vi "JSON to Variant.vi"(8 "error in (no error)":errorcluster, 10 "Variant (Data Type)":variant, 11 "JSON Value":refnum<class "JSON Value.lvclass">) -> (0 "error out":errorcluster, 2 "Variant out":variant)   [LabVIEW 2020, in "Library Commun.lvlib" / "Variant JSON.lvlib"]
doc: "Converts a JSON value object into a LabVIEW datatype.\n\nElements in the <b>Variant (Data Type)</b> are used to retrieve information from <b>JSON Value</b>.\n\nCopyright 2012 James David Powell, Shaun Rumbell and Ton Plomp\nMore information on http://lavag.org/topic/16217-cr-json-labview"
uses:
  Variant JSON.lvlib
  JSON Value/JSON Value.lvclass
  JSON Object/JSON Object.lvclass
  JSON Value/Get as JSON string.vi
  JSON Scalar/Get as I32.vi
  JSON Scalar/Get as I64.vi
  JSON Scalar/Get as U32.vi
  JSON Scalar/Get as U64.vi
  JSON Scalar/Get as SGL.vi
  JSON Scalar/Get as DBL.vi
  JSON Scalar/Get as EXT.vi
  JSON Scalar/Get as Boolean.vi
  JSON Value/Get Item by name array.vi
  JSON Scalar/Get as Path.vi
  JSON Scalar/Get as Timestamp.vi
  <userlib>/_OpenG.lib/lvdata/lvdata.llb/openg_variant.lvlib
  JSON Scalar/JSON Scalar.lvclass
  Get Polymorphic/JSON GetSet.lvlib
  <vilib>/Utility/VariantDataType/VariantType.lvlib
  support/JSON support.lvlib
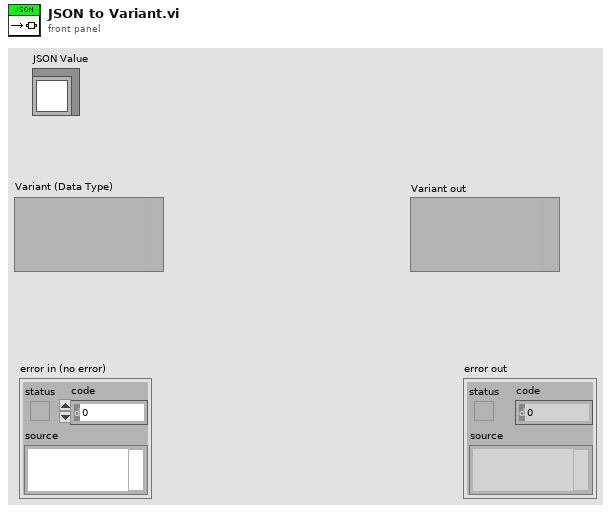
[diagram p1: front panel]
types:
  T1 = typedef "VariantType.lvlib/Type.ctl" = enum8{"Invalid Type", "Void", "I8", "I16", "I32", "I64", "U8", "U16", "U32", "U64", "Single Float", "Double Float", "Extended Float", "Single Complex", "Double Complex", "Extended Complex", "Enum U8", "Enum U16", "Enum U32", "Enum U64", "Single Float With Unit", "Double Float With Unit", "Extended Float With Unit", "Single Complex with Unit", "Double Complex with Unit", "Extended Complex with Unit", "Boolean", "String", "Path", "Picture", "Tag", "Array", "Cluster", "Variant", "LV Variant", "Waveform", "Timestamp", "Digital Waveform", "Digital Data", "ExpressData", "Refnum", "External Data", "VI", "Poly VI", "LabVIEW Class Instance", "Fixed Point"}
  T2 = cluster{"[0]":variant, "[1]":variant, "[2]":variant}
  T3 = cluster{"[0]":variant, "[1]":variant, "[2]":variant, "[3]":variant}
  T4 = cluster{"[0]":variant, "[1]":variant, "[2]":variant, "[3]":variant, "[4]":variant}
  T5 = cluster{"[0]":variant, "[1]":variant, "[2]":variant, "[3]":variant, "[4]":variant, "[5]":variant}
  T6 = cluster{"[0]":variant, "[1]":variant, "[2]":variant, "[3]":variant, "[4]":variant, "[5]":variant, "[6]":variant}
  T7 = cluster{"[0]":variant, "[1]":variant, "[2]":variant, "[3]":variant, "[4]":variant, "[5]":variant, "[6]":variant, "[7]":variant}
  T8 = cluster{"[0]":variant, "[1]":variant, "[2]":variant, "[3]":variant, "[4]":variant, "[5]":variant, "[6]":variant, "[7]":variant, "[8]":variant}
  T9 = cluster{"[0]":variant, "[1]":variant, "[2]":variant, "[3]":variant, "[4]":variant, "[5]":variant, "[6]":variant, "[7]":variant, "[8]":variant, "[9]":variant}
  T10 = typedef "VariantType.lvlib/RefnumType.ctl" = enum16{"NotARefnum", "UnknownRefnum", "Generic", "Datalog", "ByteStream", "Device", "Occurence", "TCPNetConnection", "Auto", "Menu", "Imaq", "Hardware", "DataSocket", "Visa", "IVI", "UDPNetConnection", "Notifier", "Queue", "Irda", "EventReg", "DotNet", "UserEvent", "Callback", "UNUSED_EMPTY_POSITION", "BlueToothNetConnection", "LVObjApp", "LVObjVI", "LVObjUnknown", "GenericClass", "UserDefinedRefnumTag", "DataValue", "RT FIFO", "TDMS File"}
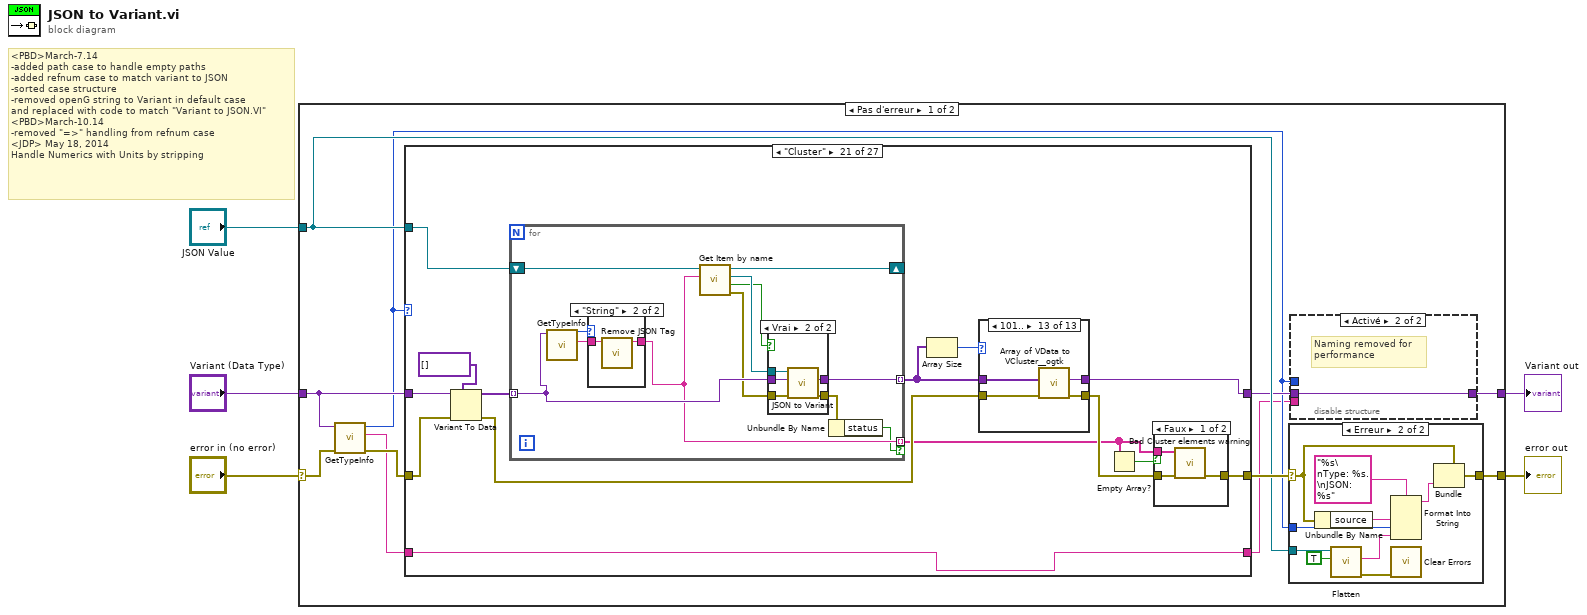
[diagram p0: block diagram]
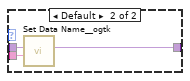
[diagram p3: hidden frame]
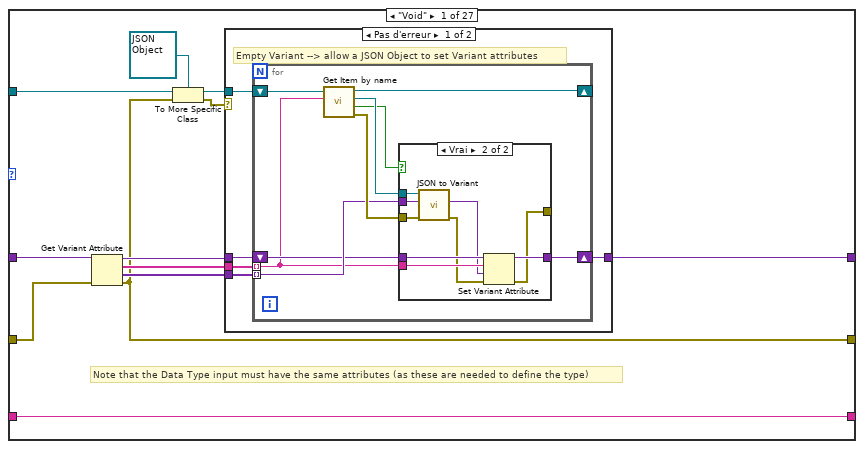
[diagram p5: hidden frame]
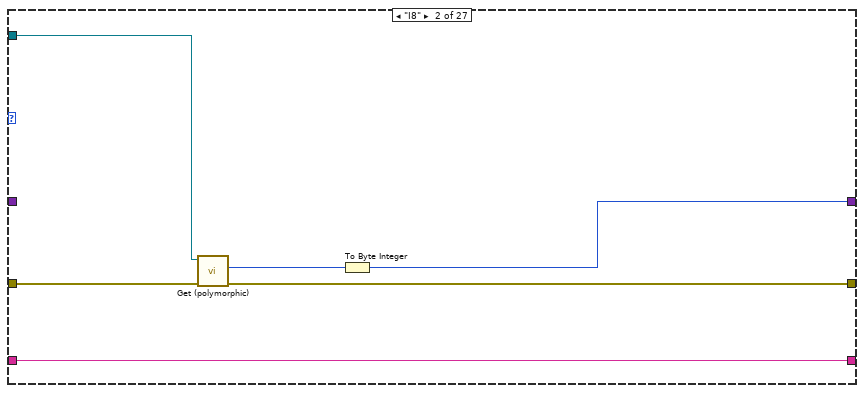
[diagram p8: hidden frame]
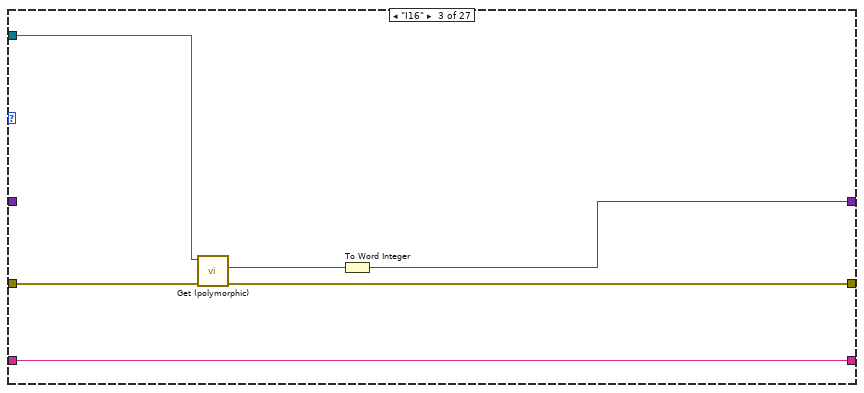
[diagram p9: hidden frame]
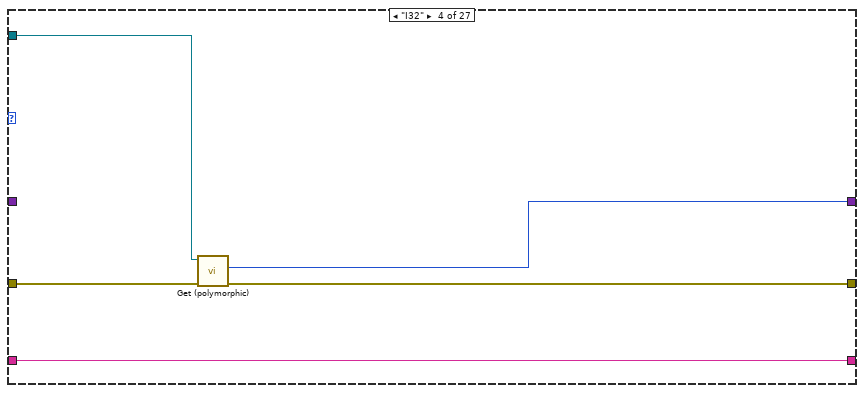
[diagram p10: hidden frame]
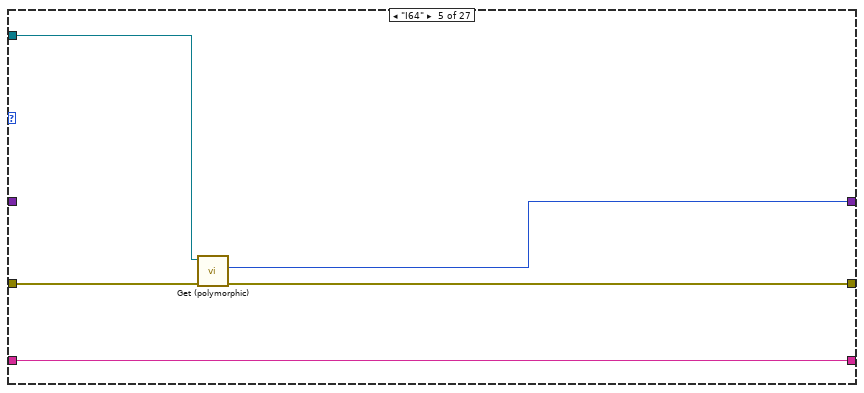
[diagram p11: hidden frame]
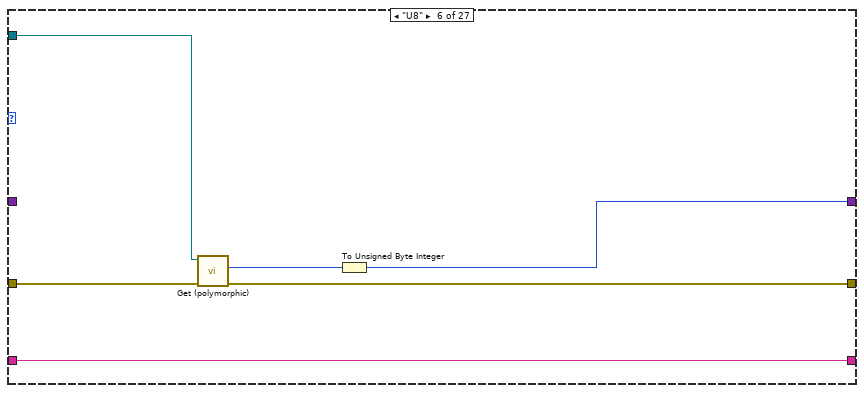
[diagram p12: hidden frame]
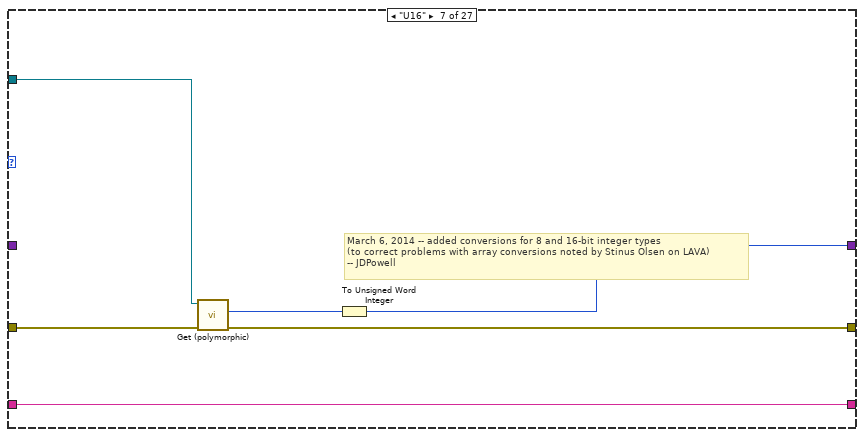
[diagram p13: hidden frame]
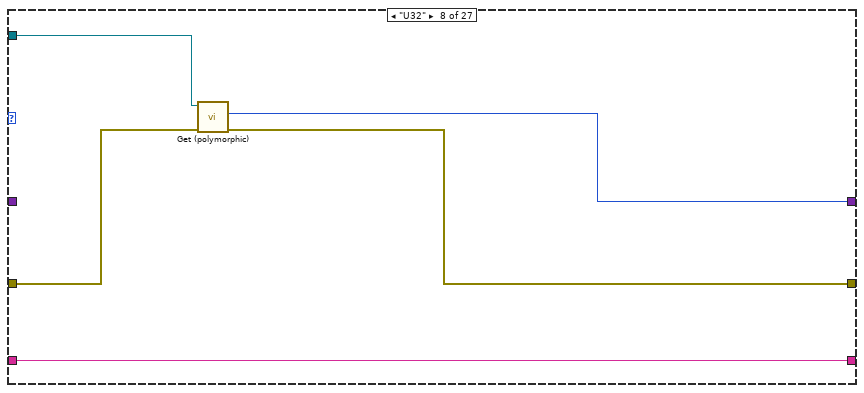
[diagram p14: hidden frame]
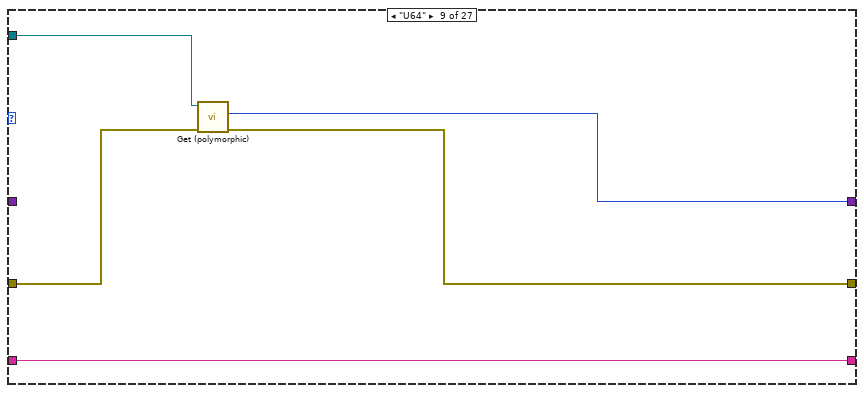
[diagram p15: hidden frame]
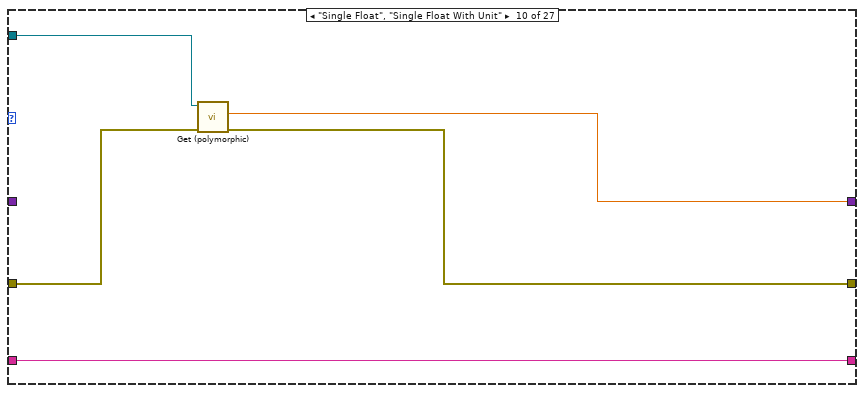
[diagram p16: hidden frame]
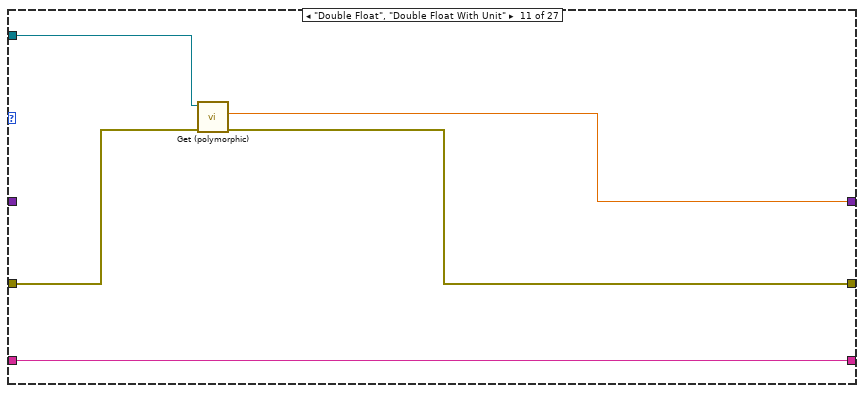
[diagram p17: hidden frame]
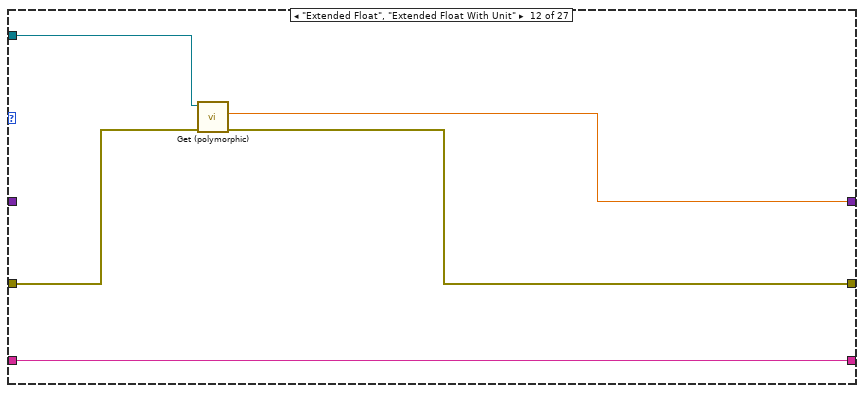
[diagram p18: hidden frame]
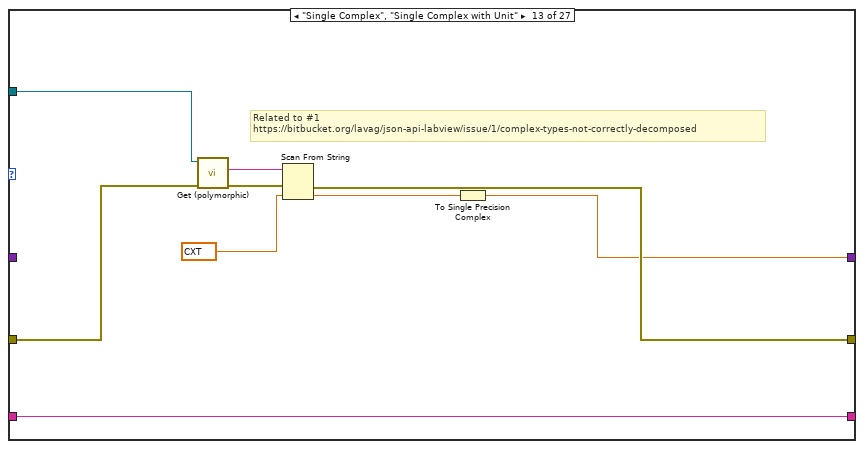
[diagram p19: hidden frame]
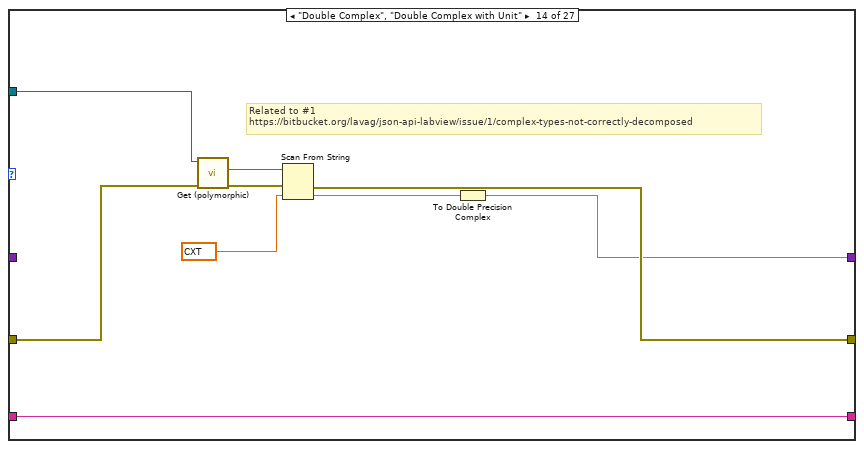
[diagram p20: hidden frame]
diagram:
  # "<PBD>March-7.14\n-added path case to handle empty paths\n-added refnum case to match variant to JSON\n-sorted case structure\n-removed openG string to Variant in default case \nand replaced with code to match \"Variant to JSON.VI\"\n<PBD>March-10.14\n-removed \"=>\" handling from refnum case\n<JDP> May 18, 2014\nHandle Numerics with Units by stripping"
  n1 = case shown="Pas d'erreur" "error in (no error)" {
    selector: "error in (no error)" -> [w10 w368]
    tunnel: [w15 w368] -> w4
    tunnel: "Variant (Data Type)" -> [w11 w367]
    tunnel: "JSON Value" -> [w14 _]
    tunnel: [w12 w367] -> w1
    frame No Error {
      n2 = call <vilib>:"GetTypeInfo.vi"("error in (no error)"=w10, "Variant"=w11) -> ("error out"=w9:errorcluster, "Name"=w7:string, "Type Enum"=w8:T1)  [unwired: 5 in, 2 out]
      n3 = case shown="\"Cluster\"" w8 {
        tunnel: w11 -> [w44 _ _ _ _ _ _ _ _ _ _ _ _ _ _ w167 _ _ _ w196 w209 w286 _ _ w304 w334 w363]
        tunnel: w9 -> [w39 w78 w84 w89 w94 w100 w106 w111 w116 w121 w126 w131 w141 w150 w158 w162 w170 w178 w192 w198 w208 w285 w291 w295 w303 _ w366]
        tunnel: [w38 w77 w83 w88 w93 w99 w105 w110 w115 w120 w125 w130 w136 w145 w153 w161 w169 w177 w191 w197 w213 w288 w290 w296 w300 w335 w361] -> w16
        tunnel: w14 -> [w48 w80 w86 w91 w96 w102 w108 w113 w118 w123 w128 w133 w142 w151 w159 w165 w172 w180 w193 w199 w212 w287 w293 w298 w302 w337 w365]
        tunnel: [w40 w76 w82 w90 w95 w98 w104 w112 w117 w122 w127 w132 w135 w144 w155 w166 w171 w179 w190 w194 w211 w280 w292 w297 w301 w336 w360] -> w13
        tunnel: w7 -> [w37 w75 w81 w87 w92 w97 w103 w109 w114 w119 w124 w129 w134 w143 w152 w160 w168 w176 w189 w195 w205 w279 w289 w294 w299 w343 w358]
        tunnel: [w37 w75 w81 w87 w92 w97 w103 w109 w114 w119 w124 w129 w134 w143 w152 w160 w168 w176 w189 w195 w205 w279 w289 w294 w299 w343 w358] -> w6
        frame "Void" {
          # "Note that the Data Type input must have the same attributes (as these are needed to define the type)"
          n4 = Get Variant Attribute(Variant=w44, error in=w39) -> (duplicate Variant=w43:variant, names=w42:string[], values=w41:variant[], error out=w38:errorcluster)  [unwired: 2 in]
          n5 = To More Specific Class(target class=refnum<class "JSON Object.lvclass"> refnum ("JSON Object in"), reference=w48, error in=w38) -> (specific class reference=w46:refnum<class "JSON Object.lvclass">, error out=w45:errorcluster)
          n6 = case shown="Pas d'erreur" w45 {
            tunnel: w46 -> [w50 _]
            tunnel: w43 -> [w51 w74]
            tunnel: w42 -> [w53 _]
            tunnel: w41 -> [w52 _]
            tunnel: [w49 w74] -> w40
            frame No Error {
              # "Empty Variant --> allow a JSON Object to set Variant attributes"
              n7 = for {
                tunnel: w53 -> [w56] mode=indexing
                tunnel: w52 -> [w58] mode=indexing
                shift-right: [w55] -> w49
                shift-left: w51 -> [w57]
                shift-right: [w54] -> _
                shift-left: w50 -> [w59]
                n8 = call-dynamic "Get Item by name.vi"("name"=w56, "JSON Object in"=w59) -> ("error out"=w62:errorcluster, "found"=w60:bool, "Value"=w61:refnum<class "JSON Value.lvclass">, "JSON Object out"=w54:refnum<class "JSON Object.lvclass">)  [unwired: 6 in]
                n9 = case shown="Vrai" w60 {
                  tunnel: w62 -> [w64 w73]
                  tunnel: [w64 w65] -> _
                  tunnel: w58 -> [_ w72]
                  tunnel: w61 -> [_ w71]
                  tunnel: w57 -> [w63 w70]
                  tunnel: w56 -> [_ w69]
                  tunnel: [w63 w68] -> w55
                  frame False {
                  }
                  frame True {
                    n10 = call "JSON to Variant.vi"("error in (no error)"=w73, "Variant (Data Type)"=w72, "JSON Value"=w71) -> ("error out"=w66:errorcluster, "Variant out"=w67:variant)  [unwired: 7 in]
                    n11 = Set Variant Attribute(Variant=w70, name=w69, value=w67, error in=w66) -> (Variant out=w68:variant, error out=w65:errorcluster)  [unwired: 1 out]
                  }
                }
              }
            }
            frame Error {
            }
          }
        }
        frame "I8" {
          n12 = call-poly "Get (polymorphic).vi"("error in (no error)"=w78, "JSON Scalar in"=w80) -> ("error out"=w77:errorcluster, "Number"=w79:i32)  [unwired: 7 in, 1 out]
          n13 = To Byte Integer(number=w79) -> (8bit integer=w76:i8)
        }
        frame "I16" {
          n14 = call-poly "Get (polymorphic).vi"("error in (no error)"=w84, "JSON Scalar in"=w86) -> ("error out"=w83:errorcluster, "Number"=w85:i32)  [unwired: 7 in, 1 out]
          n15 = To Word Integer(number=w85) -> (16bit integer=w82:i16)
        }
        frame "I32" {
          n16 = call-poly "Get (polymorphic).vi"("error in (no error)"=w89, "JSON Scalar in"=w91) -> ("error out"=w88:errorcluster, "Number"=w90:i32)  [unwired: 7 in, 1 out]
        }
        frame "I64" {
          n17 = call-poly "Get (polymorphic).vi"("error in (no error)"=w94, "JSON Scalar in"=w96) -> ("error out"=w93:errorcluster, "Number"=w95:i64)  [unwired: 7 in, 1 out]
        }
        frame "U8" {
          n18 = call-poly "Get (polymorphic).vi"("error in (no error)"=w100, "JSON Scalar in"=w102) -> ("error out"=w99:errorcluster, "Number"=w101:u32)  [unwired: 7 in, 1 out]
          n19 = To Unsigned Byte Integer(number=w101) -> (unsigned 8bit integer=w98:u8)
        }
        frame "U16" {
          # "March 6, 2014 -- added conversions for 8 and 16-bit integer types\n(to correct problems with array conversions noted by Stinus Olsen on LAVA)\n-- JDPowell"
          n20 = call-poly "Get (polymorphic).vi"("error in (no error)"=w106, "JSON Scalar in"=w108) -> ("error out"=w105:errorcluster, "Number"=w107:u32)  [unwired: 7 in, 1 out]
          n21 = To Unsigned Word Integer(number=w107) -> (unsigned 16bit integer=w104:u16)
        }
        frame "U32" {
          n22 = call-poly "Get (polymorphic).vi"("error in (no error)"=w111, "JSON Scalar in"=w113) -> ("error out"=w110:errorcluster, "Number"=w112:u32)  [unwired: 7 in, 1 out]
        }
        frame "U64" {
          n23 = call-poly "Get (polymorphic).vi"("error in (no error)"=w116, "JSON Scalar in"=w118) -> ("error out"=w115:errorcluster, "Number"=w117:u64)  [unwired: 7 in, 1 out]
        }
        frame "Single Float", "Single Float With Unit" {
          n24 = call-poly "Get (polymorphic).vi"("error in (no error)"=w121, "JSON Value in"=w123) -> ("error out"=w120:errorcluster, "Number"=w122:sgl)  [unwired: 7 in, 1 out]
        }
        frame "Double Float", "Double Float With Unit" {
          n25 = call-poly "Get (polymorphic).vi"("error in (no error)"=w126, "JSON Value in"=w128) -> ("error out"=w125:errorcluster, "Number"=w127:dbl)  [unwired: 7 in, 1 out]
        }
        frame "Extended Float", "Extended Float With Unit" {
          n26 = call-poly "Get (polymorphic).vi"("error in (no error)"=w131, "JSON Value in"=w133) -> ("error out"=w130:errorcluster, "Number"=w132:ext)  [unwired: 7 in, 1 out]
        }
        frame "Single Complex", "Single Complex with Unit" {
          # "Related to #1\nhttps://bitbucket.org/lavag/json-api-labview/issue/1/complex-types-not-correctly-decomposed"
          n27 = call-poly "Get (polymorphic).vi"("error in (no error)"=w141, "JSON Scalar in"=w142) -> ("error out"=w137:errorcluster, "LabVIEW Text"=w140:string)  [unwired: 7 in, 1 out]
          n28 = Scan From String(input string=w140, error in=w137, default 1=cxt 0.0+0.0i) -> (error out=w136:errorcluster, output 1=w138:cxt)  [unwired: 2 in, 2 out]
          n29 = To Single Precision Complex(1:w138) -> (0:w135:csg)
        }
        frame "Double Complex", "Double Complex with Unit" {
          # "Related to #1\nhttps://bitbucket.org/lavag/json-api-labview/issue/1/complex-types-not-correctly-decomposed"
          n30 = call-poly "Get (polymorphic).vi"("error in (no error)"=w150, "JSON Scalar in"=w151) -> ("error out"=w146:errorcluster, "LabVIEW Text"=w149:string)  [unwired: 7 in, 1 out]
          n31 = Scan From String(input string=w149, error in=w146, default 1=cxt 0.0+0.0i) -> (error out=w145:errorcluster, output 1=w147:cxt)  [unwired: 2 in, 2 out]
          n32 = To Double Precision Complex(1:w147) -> (0:w144:cdb)
        }
        frame "Extended Complex", "Extended Complex with Unit" {
          n33 = call-poly "Get (polymorphic).vi"("error in (no error)"=w158, "JSON Scalar in"=w159) -> ("error out"=w154:errorcluster, "LabVIEW Text"=w157:string)  [unwired: 7 in, 1 out]
          n34 = Scan From String(input string=w157, error in=w154, default 1=cxt 0.0+0.0i) -> (error out=w153:errorcluster, output 1=w155:cxt)  [unwired: 2 in, 2 out]
        }
        frame "Enum U8".."Enum U64" {
          n35 = call-poly "Get (polymorphic).vi"("error in (no error)"=w162, "JSON Scalar in"=w165) -> ("error out"=w163:errorcluster, "LabVIEW Text"=w164:string)  [unwired: 7 in, 1 out]
          n36 = call <userlib>:"Set Enum String Value__ogtk.vi"("error in (no error)"=w163, "String Value"=w164, "Default Enum Value"=w167) -> ("error out"=w161:errorcluster, "Enum"=w166:variant)  [unwired: 7 in]
        }
        frame "Boolean" {
          n37 = call-poly "Get (polymorphic).vi"("error in (no error)"=w170, "JSON Value in"=w172) -> ("error out"=w169:errorcluster, "Boolean"=w171:bool)  [unwired: 7 in, 1 out]
        }
        frame "String" {
          # "Allow marking of LabVIEW strings as representing JSON, rather than JSON strings.\nThis is to allow using Variants where some ot the subelement structure is unknown/dynamic -- JDP, April 2014"
          n38 = call "Tag for JSON Text.vi"() -> ("Tag for JSON text"=w173:string)  [unwired: 11 in]
          n39 = Match Pattern(string=w176, regular expression=w173) -> (after substring=w175:string, offset past match=w174:i32)  [unwired: 1 in, 2 out]
          n40 = case shown="0.." w174 {
            tunnel: w180 -> [w184 w188]
            tunnel: [w183 w187] -> w179
            tunnel: w178 -> [w182 w186]
            tunnel: [w181 w185] -> w177
            tunnel: w175 -> [_ _]
            frame ..-1 {
              n41 = call-poly "Get (polymorphic).vi"("error in (no error)"=w182, "JSON Scalar in"=w184) -> ("error out"=w181:errorcluster, "LabVIEW Text"=w183:string)  [unwired: 7 in, 1 out]
            }
            frame 0.. {
              n42 = call-poly "Get (polymorphic).vi"("error in (no error)"=w186, "JSON Value in"=w188) -> ("error out"=w185:errorcluster, "<JSON>"=w187:string)  [unwired: 8 in]
            }
          }
        }
        frame "Path" {
          n43 = call-poly "Get (polymorphic).vi"("error in (no error)"=w192, "JSON Scalar in"=w193) -> ("error out"=w191:errorcluster, "path"=w190:path)  [unwired: 7 in, 1 out]
        }
        frame "Array" {
          # "Dec 2015, JDP rewrite for higher speed with large arrays"
          n44 = call "Get Array as Variant.vi"("error in (no error)"=w198, "Variant (Data Type)"=w196, "JSON Value in"=w199) -> ("error out"=w197:errorcluster, "Default VData"=w194:variant)  [unwired: 7 in]
        }
        frame "Cluster" {
          n45 = Variant To Data(error in=w208, type=variant[] [], Variant=w209) -> (data=w207:variant[], error out=w206:errorcluster)
          n46 = for {
            shift-right: [w267] -> _
            shift-left: w212 -> [w268]
            tunnel: [w265] -> w202 mode=indexing
            tunnel: [w263] -> w204 mode=indexing if=w259
            tunnel: w207 -> [w264] mode=indexing
            n47 = call <vilib>:"GetTypeInfo.vi"("Variant"=w264) -> ("Name"=w258:string, "Type Enum"=w257:T1)  [unwired: 6 in, 3 out]
            n48 = case shown="\"String\"" w257 {
              tunnel: w258 -> [w269 w271]
              tunnel: [w269 w270] -> w263
              frame Default {
              }
              frame "String" {
                n49 = call "Remove JSON Tag.vi"("Name"=w271) -> ("Name (tag stripped)"=w270:string)  [unwired: 9 in, 1 out]
              }
            }
            n50 = call-dynamic "Get Item by name.vi"("name"=w263, "JSON Value In"=w268) -> ("error out"=w262:errorcluster, "found"=w260:bool, "Value"=w261:refnum<class "JSON Value.lvclass">, "JSON Value Out"=w267:refnum<class "JSON Value.lvclass">)  [unwired: 6 in]
            n51 = case shown="Vrai" w260 {
              tunnel: w262 -> [w272 w278]
              tunnel: [w272 w277] -> w266
              tunnel: w264 -> [w273 w276]
              tunnel: w261 -> [_ w275]
              tunnel: [w273 w274] -> w265
              frame False {
              }
              frame True {
                n52 = call "JSON to Variant.vi"("error in (no error)"=w278, "Variant (Data Type)"=w276, "JSON Value"=w275) -> ("error out"=w277:errorcluster, "Variant out"=w274:variant)  [unwired: 7 in]
              }
            }
            n53 = Unbundle By Name(w266) -> ("status"=w259:bool)
          }
          n54 = Array Size(array=w202) -> (size(s)=w201:i32)
          n55 = case shown="101.." w201 {
            tunnel: [variant ("VCluster") w217 w220 w223 w226 w229 w232 w235 w238 w241 w244 w247 w252] -> w211
            tunnel: [w214 w216 w219 w222 w225 w228 w231 w234 w237 w240 w243 w246 w251] -> w210
            tunnel: w206 -> [w214 w216 w219 w222 w225 w228 w231 w234 w237 w240 w243 w246 w250]
            tunnel: w202 -> [_ w218 w221 w224 w227 w230 w233 w236 w239 w242 w245 w248 w249]
            frame ..0 {
            }
            frame 1 {
              n56 = Array To Cluster(array=w218) -> (cluster=w217:cluster{"[0]":variant})
            }
            frame 2 {
              n57 = Array To Cluster(array=w221) -> (cluster=w220:cluster{"[0]":variant, "[1]":variant})
            }
            frame 3 {
              n58 = Array To Cluster(array=w224) -> (cluster=w223:T2)
            }
            frame 4 {
              n59 = Array To Cluster(array=w227) -> (cluster=w226:T3)
            }
            frame 5 {
              n60 = Array To Cluster(array=w230) -> (cluster=w229:T4)
            }
            frame 6 {
              n61 = Array To Cluster(array=w233) -> (cluster=w232:T5)
            }
            frame 7 {
              n62 = Array To Cluster(array=w236) -> (cluster=w235:T6)
            }
            frame 8 {
              n63 = Array To Cluster(array=w239) -> (cluster=w238:T7)
            }
            frame 9 {
              n64 = Array To Cluster(array=w242) -> (cluster=w241:T8)
            }
            frame 10 {
              n65 = Array To Cluster(array=w245) -> (cluster=w244:T9)
            }
            frame Default {
              n66 = call "Array of Variants to Cluster.vi"("Var"=w248) -> ("Cluster of Variants"=w247:variant)  [unwired: 10 in]
            }
            frame 101.. {
              n67 = call <userlib>:"Array of VData to VCluster__ogtk.vi"("error in (no error)"=w250, "Array"=w249) -> ("error out"=w251:errorcluster, "VCluster"=w252:variant)  [unwired: 8 in]
            }
          }
          n68 = Empty Array?(array=w204) -> (empty?=w203:bool)
          n69 = case shown="Faux" w203 {
            tunnel: [w255 w256] -> w213
            tunnel: w210 -> [w254 w256]
            tunnel: w204 -> [w253 _]
            frame False {
              n70 = call "Bad Cluster elements warning.vi"("error in (no error)"=w254, "Error items"=w253) -> ("error out"=w255:errorcluster)  [unwired: 9 in]
            }
            frame True {
            }
          }
        }
        frame "Variant", "LV Variant" {
          # "Get item inside variant, convert, and then put back in a variant"
          n71 = Variant To Data(error in=w285, type=variant, Variant=w286) -> (data=w283:variant, error out=w284:errorcluster)
          n72 = call "JSON to Variant.vi"("error in (no error)"=w284, "Variant (Data Type)"=w283, "JSON Value"=w287) -> ("error out"=w288:errorcluster, "Variant out"=w281:variant)  [unwired: 7 in]
          n73 = To Variant(anything=w281) -> (Variant=w280:variant)
        }
        frame "Waveform" {
          n74 = call "Get as Waveform.vi"("error in (no error)"=w291, "JSON Value In"=w293) -> ("error out"=w290:errorcluster, "Waveform"=w292:waveform(dbl))  [unwired: 7 in, 1 out]
        }
        frame "Timestamp" {
          n75 = call-poly "Get (polymorphic).vi"("error in (no error)"=w295, "JSON Value in"=w298) -> ("error out"=w296:errorcluster, "Time Stamp"=w297:timestamp)  [unwired: 7 in, 1 out]
        }
        frame "Refnum" {
          n76 = call-poly "Get (polymorphic).vi"("error in (no error)"=w303, "JSON Scalar in"=w302) -> ("error out"=w306:errorcluster, "LabVIEW Text"=w305:string)  [unwired: 7 in, 1 out]
          n77 = call <vilib>:"GetRefnumInfo.vi"("error in (no error)"=w306, "Variant"=w304) -> ("error out"=w307:errorcluster, "ReferenceType"=w308:T10)  [unwired: 6 in, 2 out]
          n78 = case shown="\"Visa\", \"IVI\", \"UserDefinedRefnumTag\"" w308 {
            tunnel: [w309 w318 w331] -> w301
            tunnel: w307 -> [w310 w312 w329]
            tunnel: [w310 w311 w330] -> w300
            tunnel: w305 -> [_ w313 w326]
            tunnel: w304 -> [w309 w321 w333]
            frame "NotARefnum", "UnknownRefnum" {
            }
            frame "Visa", "IVI", "UserDefinedRefnumTag" {
              n79 = Variant To Data(error in=w312, type="", Variant=w321) -> (data=w319:string, error out=w311:errorcluster)
              n80 = Scan From String(input string=w313, default 1=w319) -> (error out=w317:errorcluster, output 1=w314:string)  [unwired: 3 in, 2 out]
              n81 = Select(t="", s=w317, f=w314) -> (s? t:f=w316:string)
              n82 = To Variant(anything=w316) -> (Variant=w318:variant)
            }
            frame Default {
              w325 = 0
              n83 = Scan From String(input string=w326, default 1=w325) -> (error out=w328:errorcluster, output 1=w327:i32)  [unwired: 3 in, 2 out]
              n84 = Select(t=w325, s=w328, f=w327) -> (s? t:f=w323:i32)
              n85 = Variant To Flattened String(Variant=w333) -> (1:w332:i16[])  [unwired: 1 out]
              n86 = Type Cast(type="", x=w323) -> (*(type *) &x=w324:string)
              n87 = Flattened String To Variant(4:w329, 6:w324, 7:w332) -> (0:w330:errorcluster, 3:w331:variant)
            }
          }
        }
        frame "LabVIEW Class Instance" {
          w338 = refnum<class "JSON Value.lvclass"> refnum ("JSON Value")
          n88 = Variant To Data(type=refnum<class> refnum ("LabVIEW Object"), Variant=w334) -> (data=w339:refnum<class>, error out=w341:errorcluster)  [unwired: 1 in]
          n89 = To More Specific Class(target class=w338, reference=w339, error in=w341) -> (error out=w340:errorcluster)  [unwired: 1 out]
          n90 = case shown="Pas d'erreur" w340 {
            selector: w340 -> [w351 _]
            tunnel: w339 -> [w350 _]
            tunnel: w338 -> [w349 _]
            tunnel: w337 -> [w345 w357]
            tunnel: [w348 w354] -> w336
            tunnel: [w347 w355] -> w335
            tunnel: w334 -> [_ w353]
            frame No Error {
              # "Needed to get the wire type of the \nVariant to be the right subclass"
              # "Target is a JSON Value (or subclass), so"
              n91 = To More Specific Class(target class=w349, reference=w350, error in=w351) -> (specific class reference=w344:refnum<class "JSON Value.lvclass">, error out=w346:errorcluster)
              n92 = call-dynamic "Place in Variant.vi"("error in (no error)"=w346, "object"=w345, "wire type"=w344) -> ("error out"=w347:errorcluster, "variant (of wire type, containing object)"=w348:variant)  [unwired: 7 in]
            }
            frame Error {
              # "Fixed 3-Sep-2015 -- JDP"
              # "Try and unflatten to the supplied datatype"
              n93 = call "Get as Text.vi"("JSON Scalar in"=w357) -> ("LabVIEW Text"=w356:string)  [unwired: 8 in, 2 out]
              n94 = Variant To Flattened String(Variant=w353) -> (1:w352:i16[])  [unwired: 1 out]
              n95 = Flattened String To Variant(6:w356, 7:w352) -> (0:w355:errorcluster, 3:w354:variant)  [unwired: 1 in]
            }
          }
        }
        frame Default {
          # "Try and unflatten to the supplied data type"
          n96 = call "Get as Text.vi"("error in (no error)"=w366, "JSON Scalar in"=w365) -> ("error out"=w362:errorcluster, "LabVIEW Text"=w359:string)  [unwired: 7 in, 1 out]
          n97 = Variant To Flattened String(Variant=w363) -> (1:w364:i16[])  [unwired: 1 out]
          n98 = Flattened String To Variant(4:w362, 6:w359, 7:w364) -> (0:w361:errorcluster, 3:w360:variant)
        }
      }
      n99 = case shown="Erreur" w16 {
        selector: w16 -> [w26 w31]
        tunnel: [w26 w29] -> w15
        tunnel: w8 -> [_ w34]
        tunnel: w14 -> [_ w33]
        frame No Error {
        }
        frame Error {
          n100 = Unbundle By Name(w31) -> ("source"=w36:string)
          n101 = call-dynamic "Flatten.vi"("Pretty Print?"=TRUE, "JSON Value in"=w33) -> ("error out"=w28:errorcluster, "<JSON>"=w32:string)  [unwired: 8 in]
          n102 = Format Into String(format string="%s\nType: %s.\nJSON: %s", w36, w34, w32) -> (resulting string=w30:string)  [unwired: 2 in, 1 out]
          n103 = call <vilib>:"Clear Errors.vi"("error in (no error)"=w28) -> ()  [unwired: 5 in, 2 out]
          n104 = Bundle(cluster=w31, "source"=w30) -> (w29:errorcluster)  [unwired: 2 in]
        }
      }
      n105 = disable-structure shown="Activé" {
        disable-tunnel: w13 -> [w20 w25]
        disable-tunnel: [w19 w25] -> w12
        disable-tunnel: w8 -> [w18 _]
        disable-tunnel: w6 -> [w17 _]
        frame Disabled {
          n106 = case shown="\"Void\"" w18 {
            tunnel: w20 -> [w21 w24]
            tunnel: [w21 w23] -> w19
            tunnel: w17 -> [_ w22]
            frame "Void" {
              # "needed because\nSet Data Name will \nerror out and clear\nattributes for Void type"
            }
            frame Default {
              n107 = call <userlib>:"Set Data Name__ogtk.vi"("Data Name"=w22, "Data"=w24) -> ("Renamed Data"=w23:variant)  [unwired: 8 in, 1 out]
            }
          }
        }
        frame Enabled {
          # "Naming removed for\nperformance"
        }
      }
    }
    frame Error {
    }
  }
  "error out" <- w4
  "Variant out" <- w1
